vi "Beam Clock Ctrl.vi"(4 "Trigger Hold Off":u16, 6 "Beam Clock Config":T1, 9 "Arm":bool, 11 "Record Ticks":u16) -> (3 "Beam Clock":bool)   [LabVIEW 2014]
panel:
  # "Copyright 2014 Vidrio Technologies\nScanImage 5 software is licensed under the Apache License, Version 2.0 (the \"License\"); you may not use any files contained\nwithin the ScanImage 5 release except in compliance with the License. You may obtain a copy of the License at\n http://www.apache.org/licenses/LICENSE-2.0\nUnless required by applicable law or agreed to in writing, software distributed under the License is distributed on an\n\"AS IS\" BASIS, WITHOUT WARRANTIES OR CONDITIONS OF ANY KIND, either express or implied. See the License for the\n specific language governing permissions and limitations under the License."
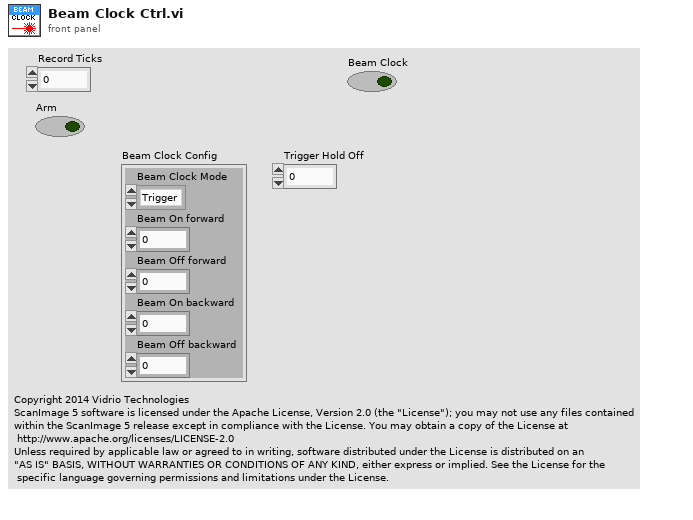
[diagram p1: front panel]
types:
  T1 = cluster{"Beam Clock Mode":enum8{"Trigger", "Toggle"}, "Beam On forward":i16, "Beam Off forward":i16, "Beam On backward":i16, "Beam Off backward":i16}
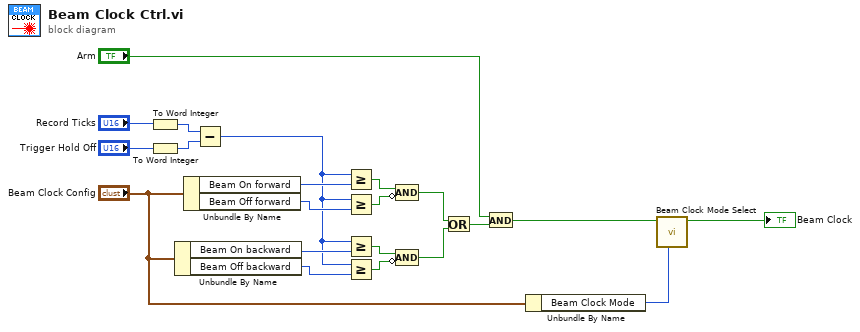
[diagram p0: block diagram]
diagram:
  n1 = To Word Integer(number="Record Ticks") -> (16bit integer=w3:i16)
  n2 = To Word Integer(number="Trigger Hold Off") -> (16bit integer=w2:i16)
  n3 = Unbundle By Name("Beam Clock Config") -> ("Beam On backward"=w19:i16, "Beam Off backward"=w18:i16)
  n4 = Unbundle By Name("Beam Clock Config") -> ("Beam On forward"=w21:i16, "Beam Off forward"=w20:i16)
  n5 = Subtract(x=w3, y=w2) -> (x-y=w1:i16)
  n6 = Greater Or Equal?(x=w1, y=w21) -> (x >= y?=w17:bool)
  n7 = Greater Or Equal?(x=w1, y=w20) -> (x >= y?=w16:bool)
  n8 = Greater Or Equal?(x=w1, y=w19) -> (x >= y?=w15:bool)
  n9 = Greater Or Equal?(x=w1, y=w18) -> (x >= y?=w14:bool)
  n10 = Compound Arithmetic op=AND(w17, invert w16) -> (w13:bool)
  n11 = Compound Arithmetic op=AND(w15, invert w14) -> (w12:bool)
  n12 = Or(x=w13, y=w12) -> (x .or. y?=w11:bool)
  n13 = And(x="Arm", y=w11) -> (x .and. y?=w9:bool)
  n14 = Unbundle By Name("Beam Clock Config") -> ("Beam Clock Mode"=w6:enum8{"Trigger", "Toggle"})
  n15 = call "Beam Clock Mode Select.vi"("Beam Clock Mode"=w6, "Beam On"=w9) -> ("Beam Clock Out"=→"Beam Clock":bool)  [unwired: 9 in]
